vi "Invert Greyscale Image In-Place.vi"(8 "error in (no error)":errorcluster, 11 "Greyscale Image to Invert in Place":T1) -> (0 "error out":errorcluster, 3 "Greyscale Image (duplicate)":T1)   [LabVIEW 2020, in "g_ar_toolkit.image.lvlib"]
uses:
  g_ar_toolkit.image.lvlib
  Greyscale Image.ctl
  g_ar_toolkit.common/g_ar_toolkit.common.lvlib
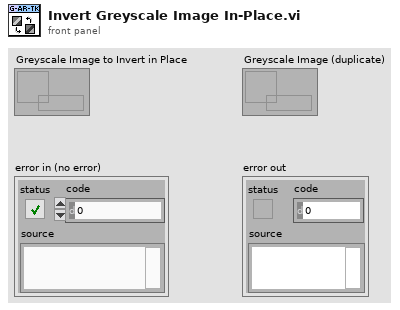
[diagram p1: front panel]
types:
  T1 = typedef "g_ar_toolkit.image.lvlib/Greyscale Image.ctl" = refnum<data-value>
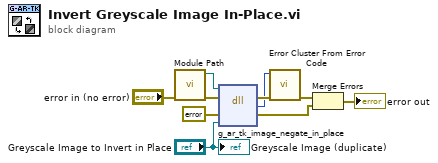
[diagram p0: block diagram]
diagram:
  n1 = call "Module Path.vi"("error in (no error)"="error in (no error)") -> ("error out"=w3:errorcluster, "Path"=w2:path)  [unwired: 9 in]
  n2 = dll-call lib="?" fn="g_ar_tk_image_negate_in_place" ("g_ar_toolkit.*.*:g_ar_tk_image_negate")(path in=w2, error in=w3, "error_cluster"=errorcluster {"status"=FALSE, "code"=0, "source"=""} ("error constant"), "EDVR image"="Greyscale Image to Invert in Place") -> (error out=w9:errorcluster, "MgErr"=w8:i32, "error_cluster"=w5:errorcluster)  [unwired: 2 in, 1 out]
  n3 = call <vilib>:"Error Cluster From Error Code.vi"("error in (no error)"=w9, "error code (0)"=w8) -> ("error out"=w7:errorcluster)  [unwired: 7 in]
  n4 = Merge Errors(w7, w5) -> (→"error out":errorcluster)
  "Greyscale Image (duplicate)" <- "Greyscale Image to Invert in Place"
